vi "Escalation Master.vi"() -> ()   [LabVIEW 2017]
uses:
  <vilib>/addons/database/Connection.llb/DB Tools Open Connec (Path).vi
  <vilib>/addons/database/NI_Database_API.lvlib
panel:
  in  "Cancel Button - Archive":bool
  in  "Update Button":bool
  in  "Get Rport":bool
  in  "EDIT":bool
  in  "String 3":string
  in  "String 2":string
  in  "String":string
  in  "Shift":string(combo)
  out "Table 2":string[][](table)
  in  "Delete":bool
  out "error out":errorcluster
  in  "error in (no error)":errorcluster
  in  "Select Stakeholder":string(combo)
  out "Table":string[][](table)
  # "Escalation Master"
  # "Designed And Developed By - Infinity Automation Systems Pvt. Ltd."
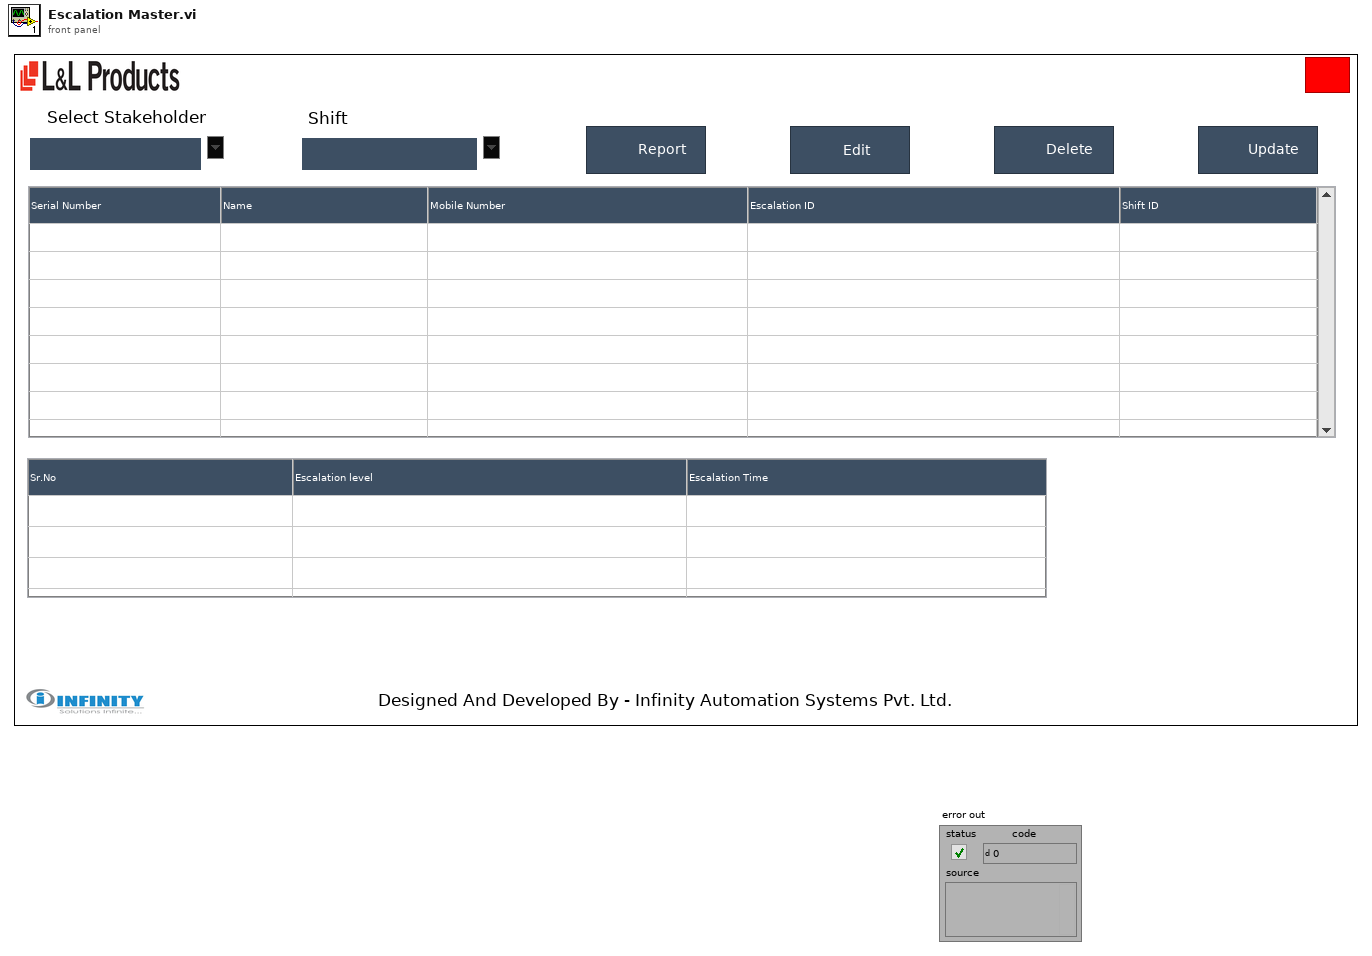
[diagram p1: front panel]
types:
  T1 = typedef "NI_Database_API.lvlib/Conn ObjectReference.ctl" = refnum<k1>
  T2 = enum32{"invalid app kind", "Development System", "Run Time System", "Student Edition", "Embedded LabVIEW", "Evaluation", "Custom"}
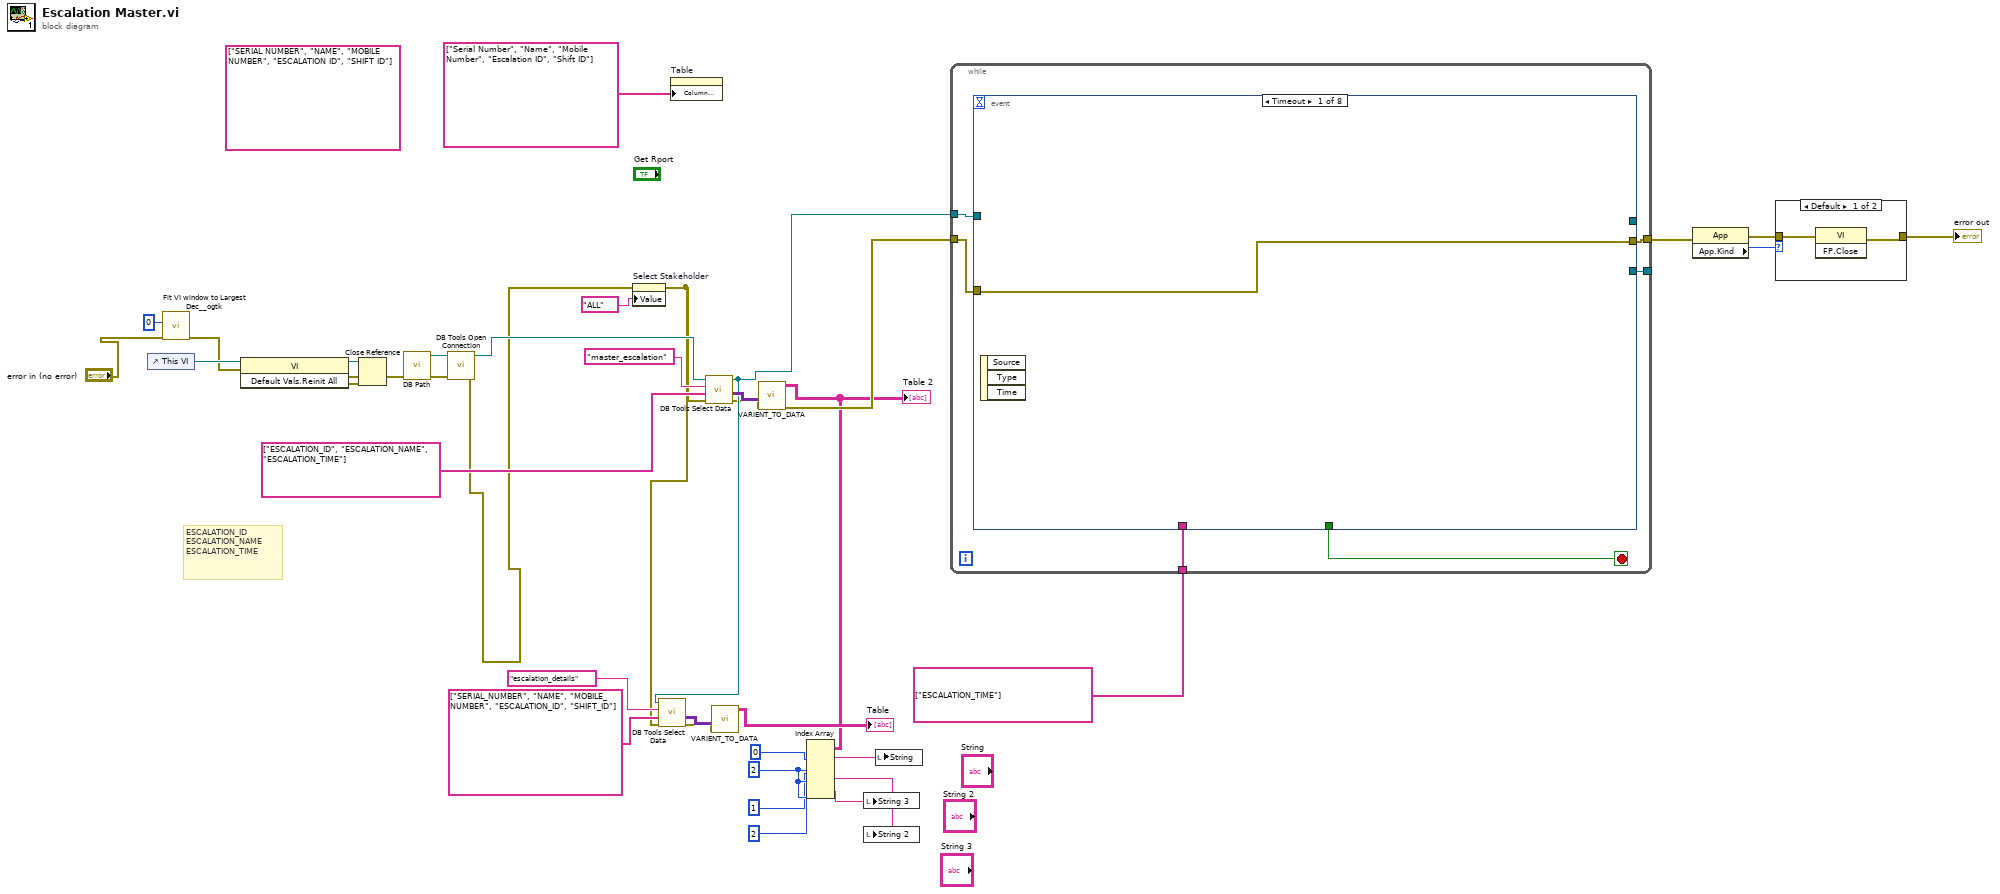
[diagram p0: block diagram]
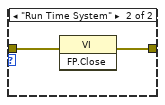
[diagram p2: hidden frame]
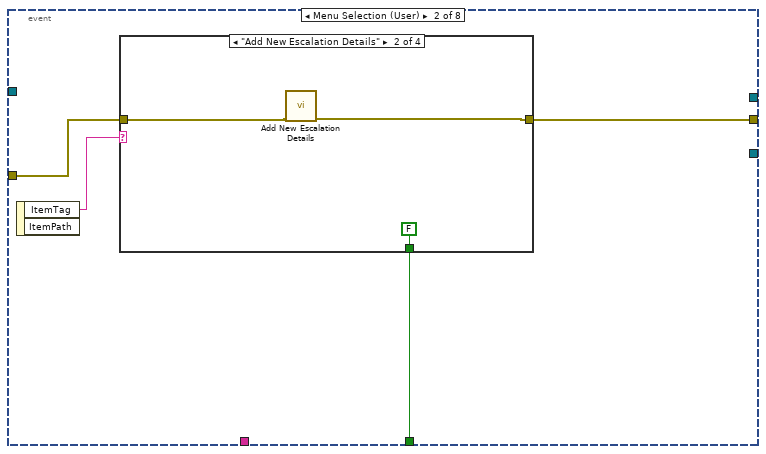
[diagram p3: hidden frame]
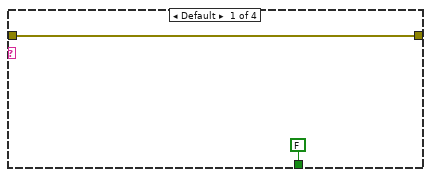
[diagram p4: hidden frame]
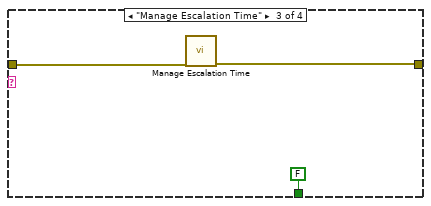
[diagram p5: hidden frame]
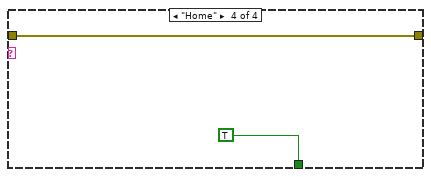
[diagram p6: hidden frame]
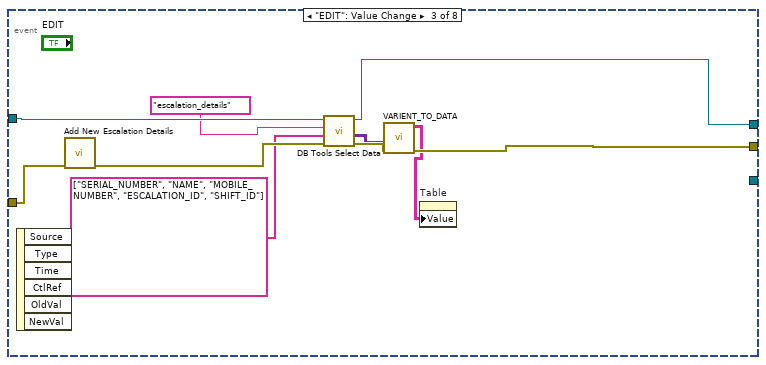
[diagram p7: hidden frame]
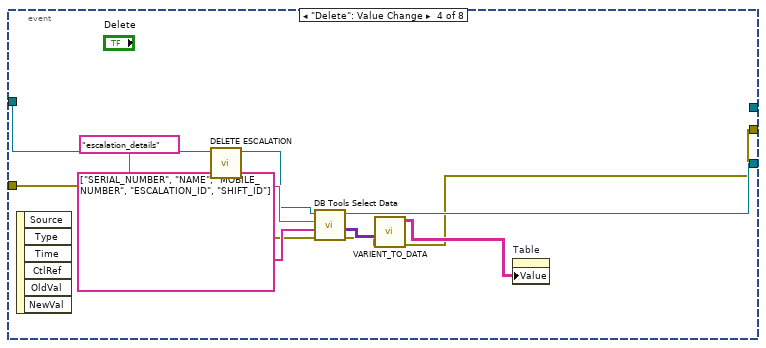
[diagram p8: hidden frame]
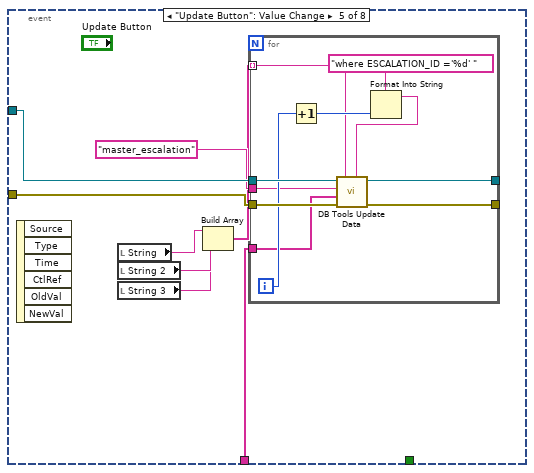
[diagram p9: hidden frame]
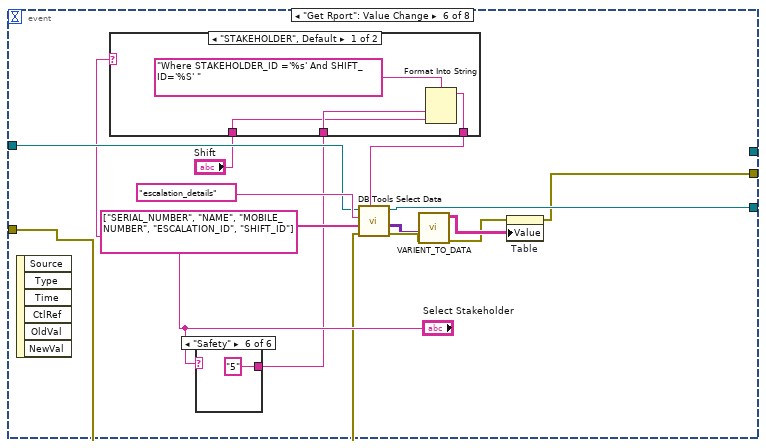
[diagram p10: hidden frame]
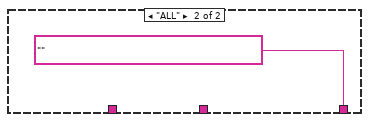
[diagram p11: hidden frame]
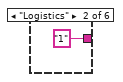
[diagram p13: hidden frame]
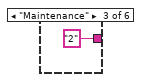
[diagram p14: hidden frame]
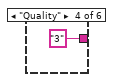
[diagram p15: hidden frame]
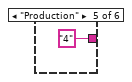
[diagram p16: hidden frame]
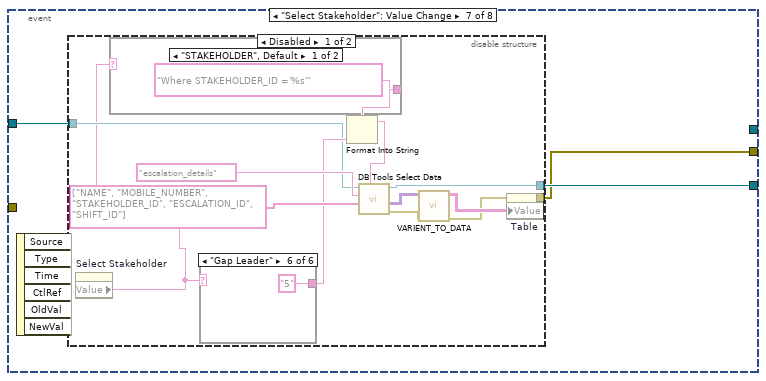
[diagram p17: hidden frame]
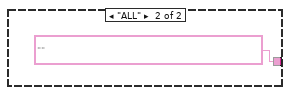
[diagram p18: hidden frame]
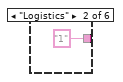
[diagram p20: hidden frame]
diagram:
  (unwired) string[] ["SERIAL NUMBER", "NAME", "MOBILE NUMBER", "ESCALATION ID", "SHIFT ID"] ("columns")
  w6 = 2 ("index (row)")
  # "ESCALATION_ID\nESCALATION_NAME\nESCALATION_TIME"
  n1 = control-ref of="This VI"() -> (w18:refnum<vi>)
  n2 = call <userlib>:"Fit VI window to Largest Dec__ogtk.vi"("error in (no error)"="error in (no error)", "border spacing (2 px)"=0) -> ("error out"=w17:errorcluster)  [unwired: 4 in, 1 out]
  n3 = invoke class="VI" method="Default Vals.Reinit All"(reference=w18, error in=w17) -> (reference out=w37:refnum<vi>, error out=w38:errorcluster)  [unwired: 1 in, 1 out]
  n4 = Close Reference(reference=w37, error in (no error)=w38) -> (error out=w28:errorcluster)
  n5 = call "DB Path.vi"("error in"=w28) -> ("error out"=w30:errorcluster, "DB Path"=w29:path)  [unwired: 9 in]
  n6 = call-poly <vilib>:"DB Tools Open Connection.vi"("error in (no error)"=w30, "connection information"=w29) -> ("error out"=w14:errorcluster, "connection reference"=w27:T1)  [unwired: 6 in]
  n7 = property on="Select Stakeholder" class="CmbBox"(error in=w14, "Value"="ALL" ("Select Stakeholder")) -> (error out=w13:errorcluster)  [unwired: 1 in, 1 out]
  n8 = property on="Table" class="Tbl (strict)"("Column Headers[]"=string[] ["Serial Number", "Name", "Mobile Number", "Escalation ID", "Shift ID"] ("columns")) -> ()  [unwired: 2 in, 2 out]
  n9 = call <vilib>:"DB Tools Select Data.vi"("error in (no error)"=w13, "columns"=string[] ["ESCALATION_ID", "ESCALATION_NAME", "ESCALATION_TIME"], "table"="master_escalation", "connection reference"=w27) -> ("error out"=w15:errorcluster, "data"=w32:variant[][], "connection reference out"=w22:T1)  [unwired: 2 in]
  n10 = call <vilib>:"DB Tools Select Data.vi"("error in (no error)"=w13, "columns"=string[] ["SERIAL_NUMBER", "NAME", "MOBILE_NUMBER", "ESCALATION_ID", "SHIFT_ID"], "table"="escalation_details", "connection reference"=w22) -> ("error out"=w23:errorcluster, "data"=w24:variant[][])  [unwired: 2 in, 1 out]
  n11 = call "VARIENT_TO_DATA.vi"("data"=w24, "error in (no error)"=w23) -> ("Table"=→"Table":string[][])  [unwired: 7 in, 1 out]
  n12 = call "VARIENT_TO_DATA.vi"("data"=w32, "error in (no error)"=w15) -> ("Table"=w7:string[][], "error out"=w31:errorcluster)  [unwired: 7 in]
  "Table 2" <- w7
  n13 = Index Array(array=w7, index (row) #1=0 ("index (row)"), index (col) #1=w6, index (row) #2=1 ("index (row)"), index (col) #2=w6, index (row) #3=2 ("index (row)"), index (col) #3=w6) -> (element #1=w2:string, element #2=w3:string, element #3=w1:string)
  n14 = local write "String 3"(w1) -> ()
  n15 = local write "String 2"(w3) -> ()
  n16 = local write "String"(w2) -> ()
  n17 = while {
    tunnel: w31 -> [w44]
    tunnel: [w40] -> w33
    tunnel: w22 -> [w42]
    tunnel: [w41] -> _
    tunnel: string[] ["ESCALATION_TIME"] ("columns") -> [w39]
    stop <- w43 stop-if-true
    n18 = event shown="[0] Timeout" {
      selector: _ -> [_ _ _ _ _ _ _ _]
      dyn-events: _ -> [_ _ _ _ _ _ _ _]
      timeout: _ -> [_ _ _ _ _ _ _ _]
      tunnel: w44 -> [w45 w46 w69 w80 w87 w100 _ _]
      tunnel: [_ w48 _ _ _ _ _ TRUE] -> w43
      tunnel: w42 -> [_ _ w64 w79 w88 w108 w126 _]
      tunnel: [_ _ w63 _ _ _ _ _] -> _
      tunnel: [_ _ _ w73 _ w107 w125 _] -> w41
      tunnel: [w45 w47 w65 w70 _ w105 w124 _] -> w40
      tunnel: w39 -> [_ _ _ _ w85 _ _ _]
      event Timeout {
        n19 = event-data() -> ()  [unwired: 1 in, 3 out]
      }
      event Menu Selection (User) {
        n20 = event-data() -> ("ItemTag"=w49:string)  [unwired: 1 in, 1 out]
        n21 = case shown="\"Add New Escalation Details\"" w49 {
          tunnel: [FALSE FALSE FALSE TRUE] -> w48
          tunnel: [w50 w53 w56 w58] -> w47
          tunnel: w46 -> [w50 w54 w57 w58]
          frame Default {
          }
          frame "Add New Escalation Details" {
            n22 = call "Add New Escalation Details.vi"("error in (no error)"=w54) -> ("error out"=w53:errorcluster)  [unwired: 10 in]
          }
          frame "Manage Escalation Time" {
            n23 = call "Manage Escalation Time.vi"("error in (no error)"=w57) -> ("error out"=w56:errorcluster)  [unwired: 10 in]
          }
          frame "Home" {
          }
        }
      }
      event "EDIT": Value Change {
        n24 = event-data() -> ()  [unwired: 1 in, 6 out]
        n25 = call "Add New Escalation Details.vi"("error in (no error)"=w69) -> ("error out"=w66:errorcluster)  [unwired: 10 in]
        n26 = call <vilib>:"DB Tools Select Data.vi"("error in (no error)"=w66, "columns"=string[] ["SERIAL_NUMBER", "NAME", "MOBILE_NUMBER", "ESCALATION_ID", "SHIFT_ID"], "table"="escalation_details", "connection reference"=w64) -> ("error out"=w68:errorcluster, "data"=w67:variant[][], "connection reference out"=w63:T1)  [unwired: 2 in]
        n27 = call "VARIENT_TO_DATA.vi"("data"=w67, "error in (no error)"=w68) -> ("Table"=w61:string[][], "error out"=w65:errorcluster)  [unwired: 7 in]
        n28 = property on="Table" class="Tbl (strict)"("Value"=w61) -> ()  [unwired: 2 in, 2 out]
      }
      event "Delete": Value Change {
        n29 = event-data() -> ()  [unwired: 1 in, 6 out]
        n30 = call "DELETE ESCALATION.vi"("error in (no error)"=w80, "connection reference"=w79) -> ("error out"=w71:errorcluster, "connection reference out"=w74:T1)  [unwired: 8 in]
        n31 = call <vilib>:"DB Tools Select Data.vi"("error in (no error)"=w71, "columns"=string[] ["SERIAL_NUMBER", "NAME", "MOBILE_NUMBER", "ESCALATION_ID", "SHIFT_ID"], "table"="escalation_details", "connection reference"=w74) -> ("error out"=w77:errorcluster, "data"=w78:variant[][], "connection reference out"=w73:T1)  [unwired: 2 in]
        n32 = call "VARIENT_TO_DATA.vi"("data"=w78, "error in (no error)"=w77) -> ("Table"=w72:string[][], "error out"=w70:errorcluster)  [unwired: 7 in]
        n33 = property on="Table" class="Tbl (strict)"("Value"=w72) -> ()  [unwired: 2 in, 2 out]
      }
      event "Update Button": Value Change {
        n34 = event-data() -> ()  [unwired: 1 in, 6 out]
        n35 = local read "String"() -> (w84:string)
        n36 = local read "String 2"() -> (w83:string)
        n37 = local read "String 3"() -> (w82:string)
        n38 = Build Array(w84, w83, w82) -> (w81:string[])
        n39 = for {
          tunnel: "master_escalation" ("table") -> [w90]
          tunnel: w85 -> [w91]
          tunnel: w88 -> [w97]
          tunnel: [w96] -> _
          tunnel: w87 -> [w99]
          tunnel: [w98] -> _
          tunnel: w81 -> [w89] mode=indexing
          i -> [w93]
          n40 = Increment(x=w93) -> (x+1=w92:i32)
          n41 = Format Into String(format string="where ESCALATION_ID ='%d' ", w92) -> (resulting string=w95:string)  [unwired: 2 in, 1 out]
          n42 = call <vilib>:"DB Tools Update Data.vi"("condition"=w95, "data"=w89, "error in (no error)"=w99, "columns"=w91, "table"=w90, "connection reference"=w97) -> ("error out"=w98:errorcluster, "connection reference out"=w96:T1)  [unwired: 4 in]
        }
      }
      event "Get Rport": Value Change {
        n43 = event-data() -> ()  [unwired: 1 in, 6 out]
        n44 = case shown="\"Safety\"" "Select Stakeholder" {
          tunnel: [_ "1" "2" "3" "4" "5"] -> w103
          frame "False", Default {
          }
          frame "Logistics" {
          }
          frame "Maintenance" {
          }
          frame "Quality" {
          }
          frame "Production" {
          }
          frame "Safety" {
          }
        }
        n45 = case shown="\"STAKEHOLDER\", Default" "Select Stakeholder" {
          tunnel: w103 -> [w116 _]
          tunnel: "Shift" -> [w115 _]
          tunnel: [w114 ""] -> w101
          frame "STAKEHOLDER", Default {
            n46 = Format Into String(format string="Where STAKEHOLDER_ID ='%s' And SHIFT_ID='%S' ", w116, w115) -> (resulting string=w114:string)  [unwired: 2 in, 1 out]
          }
          frame "ALL" {
          }
        }
        n47 = call <vilib>:"DB Tools Select Data.vi"("condition"=w101, "error in (no error)"=w100, "columns"=string[] ["SERIAL_NUMBER", "NAME", "MOBILE_NUMBER", "ESCALATION_ID", "SHIFT_ID"], "table"="escalation_details", "connection reference"=w108) -> ("error out"=w113:errorcluster, "data"=w112:variant[][], "connection reference out"=w107:T1)  [unwired: 1 in]
        n48 = call "VARIENT_TO_DATA.vi"("data"=w112, "error in (no error)"=w113) -> ("Table"=w111:string[][], "error out"=w106:errorcluster)  [unwired: 7 in]
        n49 = property on="Table" class="Tbl (strict)"(error in=w106, "Value"=w111) -> (error out=w105:errorcluster)  [unwired: 1 in, 1 out]
      }
      event "Select Stakeholder": Value Change {
        n50 = event-data() -> ()  [unwired: 1 in, 6 out]
        n51 = disable-structure shown="Disabled" {
          disable-tunnel: w126 -> [w131 _]
          disable-tunnel: [w130 _] -> w125
          disable-tunnel: [w128 _] -> w124
          frame Disabled {
            n52 = property on="Select Stakeholder" class="CmbBox"() -> ("Value"=w127:string)  [unwired: 2 in, 2 out]
            n53 = case shown="\"STAKEHOLDER\", Default" w127 {
              tunnel: ["Where STAKEHOLDER_ID ='%s'" ""] -> w134
              frame "STAKEHOLDER", Default {
              }
              frame "ALL" {
              }
            }
            n54 = case shown="\"Gap Leader\"" w127 {
              tunnel: [_ "1" "2" "3" "4" "5"] -> w132
              frame "False", Default {
              }
              frame "Logistics" {
              }
              frame "Maintenance" {
              }
              frame "Quality" {
              }
              frame "Production" {
              }
              frame "Gap Leader" {
              }
            }
            n55 = Format Into String(format string=w134, w132) -> (resulting string=w133:string)  [unwired: 2 in, 1 out]
            n56 = call <vilib>:"DB Tools Select Data.vi"("condition"=w133, "columns"=string[] ["NAME", "MOBILE_NUMBER", "STAKEHOLDER_ID", "ESCALATION_ID", "SHIFT_ID"], "table"="escalation_details", "connection reference"=w131) -> ("error out"=w139:errorcluster, "data"=w138:variant[][], "connection reference out"=w130:T1)  [unwired: 2 in]
            n57 = call "VARIENT_TO_DATA.vi"("error in (no error)"=w139, "data"=w138) -> ("error out"=w129:errorcluster, "Table"=w137:string[][])  [unwired: 8 in]
            n58 = property on="Table" class="Tbl (strict)"(error in=w129, "Value"=w137) -> (error out=w128:errorcluster)  [unwired: 1 in, 1 out]
          }
          frame Enabled {
          }
        }
      }
      event "Cancel Button - Archive": Value Change {
        n59 = event-data() -> ()  [unwired: 1 in, 6 out]
      }
    }
  }
  n60 = property class="App"(error in=w33) -> (error out=w35:errorcluster, "App.Kind"=w36:T2)  [unwired: 1 in, 1 out]
  n61 = case shown="Default" w36 {
    tunnel: w35 -> [w149 w151]
    tunnel: [w148 w150] -> w34
    frame Default {
      n62 = invoke class="VI" method="FP.Close"(error in=w149) -> (error out=w148:errorcluster)  [unwired: 2 in, 2 out]
    }
    frame "Run Time System" {
      n63 = invoke class="VI" method="FP.Close"(error in=w151) -> (error out=w150:errorcluster)  [unwired: 2 in, 2 out]
    }
  }
  "error out" <- w34
